vi "PicoScope6000aExampleBlock.vi"() -> ()   [LabVIEW 2016]
uses:
  <vilib>/Waveform/DWDTOps.llb/DWDT Analog to Digital.vi
  PicoScope6000aLib/PicoScope6000aAnalogChannelSettings.ctl
  PicoScope6000aLib/PicoScope6000aDigitalChannelSettings.ctl
panel:
  in  "Digital Channels":T1={"Port 0 Settings "={"Enabled"=FALSE, "Hysteresis"=3, "Threshold Level (Volts)"=[1.0, 1.0, 1.0, 1.0, 1.0, 1.0, 1.0, 1.0]}, "Port 1 Settings"={"Enabled"=FALSE, "Hysteresis"=3, "Threshold Level (Volts)"=[1.0, 1.0, 1.0, 1.0, 1.0, 1.0, 1.0, 1.0]}} {"Port 1 Settings"."Threshold Level (Volts)" format="%#_4p"; "Port 1 Settings"."Hysteresis" items=["PICO_VERY_HIGH_400MV", "PICO_HIGH_200MV", "PICO_NORMAL_100MV", "PICO_LOW_50MV"]; "Port 0 Settings"."Threshold Level (Volts)" format="%#_4p"; "Port 0 Settings"."Hysteresis" items=["PICO_VERY_HIGH_400MV", "PICO_HIGH_200MV", "PICO_NORMAL_100MV", "PICO_LOW_50MV"]}
  in  "Channels":T2={"Channel A Settings "={"Enabled"=TRUE, "Coupling"=1, "Range"=0, "Analogue Offset"=0.0, "BandWidth"=0}, "Channel B Settings "={"Enabled"=FALSE, "Coupling"=1, "Range"=0, "Analogue Offset"=0.0, "BandWidth"=0}, "Channel C Settings "={"Enabled"=FALSE, "Coupling"=1, "Range"=0, "Analogue Offset"=0.0, "BandWidth"=0}, "Channel D Settings "={"Enabled"=FALSE, "Coupling"=1, "Range"=0, "Analogue Offset"=0.0, "BandWidth"=0}, "Channel E Settings "={"Enabled"=FALSE, "Coupling"=1, "Range"=0, "Analogue Offset"=0.0, "BandWidth"=0}, "Channel F Settings "={"Enabled"=FALSE, "Coupling"=1, "Range"=0, "Analogue Offset"=0.0, "BandWidth"=0}, "Channel G Settings "={"Enabled"=FALSE, "Coupling"=1, "Range"=0, "Analogue Offset"=0.0, "BandWidth"=0}, "Channel H Settings "={"Enabled"=FALSE, "Coupling"=1, "Range"=0, "Analogue Offset"=0.0, "BandWidth"=0}} {"Channel H Settings"."BandWidth" items=["Full"=0, "100kHz"=100000, "20kHz"=200000, "1MHz"=1000000, "20MHz"=20000000, "25MHz"=25000000, "50MHz"=50000000, "200MHz"=200000000, "250MHz"=250000000, "500MHz"=500000000]; "Channel H Settings"."Range" items=["10mV"=0, "20mV"=1, "50mV"=2, "100mV"=3, "200mV"=4, "500mV"=5, "1V"=6, "2V"=7, "5V"=8, "10V"=9, "20V"=10, "50V"=11, "100V"=12, "200V"=13, "x10_Probe_100mV"=32, "x10_Probe_200mV"=33, "x10_Probe_500mV"=34, "x10_Probe_1V"=35, "x10_Probe_2V"=36, "x10_Probe_5V"=37, "x10_Probe_10V"=38, "x10_Probe_20V"=39, "x10_Probe_50V"=40, "x10_Probe_100V"=41, "x10_Probe_200V"=42, "x10_Probe_500V"=43, "CURRENT_CLAMP_60A_2A"=10500, "CURRENT_CLAMP_60A_5A"=10501, "CURRENT_CLAMP_60A_10A"=10502, "CURRENT_CLAMP_60A_20A"=10503, "CURRENT_CLAMP_60A_50A"=10504, "CURRENT_CLAMP_60A_60A"=10505, "CURRENT_CLAMP_60A_V2_0_5A"=10600, "CURRENT_CLAMP_60A_V2_1A"=10601, "CURRENT_CLAMP_60A_V2_2A"=10602, "CURRENT_CLAMP_60A_V2_5A"=10603, "CURRENT_CLAMP_60A_V2_10A"=10604, "CURRENT_CLAMP_60A_V2_20A"=10605, "CURRENT_CLAMP_60A_V2_50A"=10606, "CURRENT_CLAMP_60A_V2_60A"=10607, "RESISTANCE_LEAD_NEG5_TO_20OHM"=7000, "RESISTANCE_LEAD_NEG50_TO_200OHM"=7001, "RESISTANCE_LEAD_NEG500_TO_2KOHM"=7002, "RESISTANCE_LEAD_NEG5K_TO_20KOHM"=7003, "RESISTANCE_LEAD_NEG50K_TO_LEAD_200KOHM"=7004, "RESISTANCE_LEAD_NEG500K_TO_LEAD_2MOHM"=7005, "RESISTANCE_LEAD_DIODE_TEST"=7006, "HT_NEG3_TO_5KV"=8950, "HT_NEG3_TO_10KV"=8951, "HT_NEG5_TO_20KV"=8952, "HT_NEG5_TO_50KV"=8953, "HT_NEG5_TO_100KV"=8954, "HT_NEG3_TO_5KV_INVERTED"=8955, "HT_NEG3_TO_10KV_INVERTED"=8956, "HT_NEG5_TO_20KV_INVERTED"=8957, "HT_NEG5_TO_50KV_INVERTED"=8958, "HT_NEG5_TO_100KV_INVERTED"=8959, "TEMPERATURE_NEG50_TO_150DEGC"=9000, "PRESSURE_SENSOR_-100k-150k_PASCALS"=9100, "PRESSURE_SENSOR_-100k_TO_400k_PASCALS"=9101, "PRESSURE_SENSOR_-200k_TO_800k_PASCALS"=9102, "PRESSURE_SENSOR_-400k_TO_1600k_PASCALS"=9103, "PRESSURE_SENSOR_-400k_TO_3400k_PASCALS"=9104, "PRESSURE_SENSOR_-150k_TO_1350k_PASCALS"=9105]; "Channel H Settings"."Coupling" items=["AC"=0, "DC 1M Ohm"=1, "DC 50 Ohm"=50]; "Channel G Settings"."BandWidth" items=["Full"=0, "100kHz"=100000, "20kHz"=200000, "1MHz"=1000000, "20MHz"=20000000, "25MHz"=25000000, "50MHz"=50000000, "200MHz"=200000000, "250MHz"=250000000, "500MHz"=500000000]; "Channel G Settings"."Range" items=["10mV"=0, "20mV"=1, "50mV"=2, "100mV"=3, "200mV"=4, "500mV"=5, "1V"=6, "2V"=7, "5V"=8, "10V"=9, "20V"=10, "50V"=11, "100V"=12, "200V"=13, "x10_Probe_100mV"=32, "x10_Probe_200mV"=33, "x10_Probe_500mV"=34, "x10_Probe_1V"=35, "x10_Probe_2V"=36, "x10_Probe_5V"=37, "x10_Probe_10V"=38, "x10_Probe_20V"=39, "x10_Probe_50V"=40, "x10_Probe_100V"=41, "x10_Probe_200V"=42, "x10_Probe_500V"=43, "CURRENT_CLAMP_60A_2A"=10500, "CURRENT_CLAMP_60A_5A"=10501, "CURRENT_CLAMP_60A_10A"=10502, "CURRENT_CLAMP_60A_20A"=10503, "CURRENT_CLAMP_60A_50A"=10504, "CURRENT_CLAMP_60A_60A"=10505, "CURRENT_CLAMP_60A_V2_0_5A"=10600, "CURRENT_CLAMP_60A_V2_1A"=10601, "CURRENT_CLAMP_60A_V2_2A"=10602, "CURRENT_CLAMP_60A_V2_5A"=10603, "CURRENT_CLAMP_60A_V2_10A"=10604, "CURRENT_CLAMP_60A_V2_20A"=10605, "CURRENT_CLAMP_60A_V2_50A"=10606, "CURRENT_CLAMP_60A_V2_60A"=10607, "RESISTANCE_LEAD_NEG5_TO_20OHM"=7000, "RESISTANCE_LEAD_NEG50_TO_200OHM"=7001, "RESISTANCE_LEAD_NEG500_TO_2KOHM"=7002, "RESISTANCE_LEAD_NEG5K_TO_20KOHM"=7003, "RESISTANCE_LEAD_NEG50K_TO_LEAD_200KOHM"=7004, "RESISTANCE_LEAD_NEG500K_TO_LEAD_2MOHM"=7005, "RESISTANCE_LEAD_DIODE_TEST"=7006, "HT_NEG3_TO_5KV"=8950, "HT_NEG3_TO_10KV"=8951, "HT_NEG5_TO_20KV"=8952, "HT_NEG5_TO_50KV"=8953, "HT_NEG5_TO_100KV"=8954, "HT_NEG3_TO_5KV_INVERTED"=8955, "HT_NEG3_TO_10KV_INVERTED"=8956, "HT_NEG5_TO_20KV_INVERTED"=8957, "HT_NEG5_TO_50KV_INVERTED"=8958, "HT_NEG5_TO_100KV_INVERTED"=8959, "TEMPERATURE_NEG50_TO_150DEGC"=9000, "PRESSURE_SENSOR_-100k-150k_PASCALS"=9100, "PRESSURE_SENSOR_-100k_TO_400k_PASCALS"=9101, "PRESSURE_SENSOR_-200k_TO_800k_PASCALS"=9102, "PRESSURE_SENSOR_-400k_TO_1600k_PASCALS"=9103, "PRESSURE_SENSOR_-400k_TO_3400k_PASCALS"=9104, "PRESSURE_SENSOR_-150k_TO_1350k_PASCALS"=9105]; "Channel G Settings"."Coupling" items=["AC"=0, "DC 1M Ohm"=1, "DC 50 Ohm"=50]; "Channel F Settings"."BandWidth" items=["Full"=0, "100kHz"=100000, "20kHz"=200000, "1MHz"=1000000, "20MHz"=20000000, "25MHz"=25000000, "50MHz"=50000000, "200MHz"=200000000, "250MHz"=250000000, "500MHz"=500000000]; "Channel F Settings"."Range" items=["10mV"=0, "20mV"=1, "50mV"=2, "100mV"=3, "200mV"=4, "500mV"=5, "1V"=6, "2V"=7, "5V"=8, "10V"=9, "20V"=10, "50V"=11, "100V"=12, "200V"=13, "x10_Probe_100mV"=32, "x10_Probe_200mV"=33, "x10_Probe_500mV"=34, "x10_Probe_1V"=35, "x10_Probe_2V"=36, "x10_Probe_5V"=37, "x10_Probe_10V"=38, "x10_Probe_20V"=39, "x10_Probe_50V"=40, "x10_Probe_100V"=41, "x10_Probe_200V"=42, "x10_Probe_500V"=43, "CURRENT_CLAMP_60A_2A"=10500, "CURRENT_CLAMP_60A_5A"=10501, "CURRENT_CLAMP_60A_10A"=10502, "CURRENT_CLAMP_60A_20A"=10503, "CURRENT_CLAMP_60A_50A"=10504, "CURRENT_CLAMP_60A_60A"=10505, "CURRENT_CLAMP_60A_V2_0_5A"=10600, "CURRENT_CLAMP_60A_V2_1A"=10601, "CURRENT_CLAMP_60A_V2_2A"=10602, "CURRENT_CLAMP_60A_V2_5A"=10603, "CURRENT_CLAMP_60A_V2_10A"=10604, "CURRENT_CLAMP_60A_V2_20A"=10605, "CURRENT_CLAMP_60A_V2_50A"=10606, "CURRENT_CLAMP_60A_V2_60A"=10607, "RESISTANCE_LEAD_NEG5_TO_20OHM"=7000, "RESISTANCE_LEAD_NEG50_TO_200OHM"=7001, "RESISTANCE_LEAD_NEG500_TO_2KOHM"=7002, "RESISTANCE_LEAD_NEG5K_TO_20KOHM"=7003, "RESISTANCE_LEAD_NEG50K_TO_LEAD_200KOHM"=7004, "RESISTANCE_LEAD_NEG500K_TO_LEAD_2MOHM"=7005, "RESISTANCE_LEAD_DIODE_TEST"=7006, "HT_NEG3_TO_5KV"=8950, "HT_NEG3_TO_10KV"=8951, "HT_NEG5_TO_20KV"=8952, "HT_NEG5_TO_50KV"=8953, "HT_NEG5_TO_100KV"=8954, "HT_NEG3_TO_5KV_INVERTED"=8955, "HT_NEG3_TO_10KV_INVERTED"=8956, "HT_NEG5_TO_20KV_INVERTED"=8957, "HT_NEG5_TO_50KV_INVERTED"=8958, "HT_NEG5_TO_100KV_INVERTED"=8959, "TEMPERATURE_NEG50_TO_150DEGC"=9000, "PRESSURE_SENSOR_-100k-150k_PASCALS"=9100, "PRESSURE_SENSOR_-100k_TO_400k_PASCALS"=9101, "PRESSURE_SENSOR_-200k_TO_800k_PASCALS"=9102, "PRESSURE_SENSOR_-400k_TO_1600k_PASCALS"=9103, "PRESSURE_SENSOR_-400k_TO_3400k_PASCALS"=9104, "PRESSURE_SENSOR_-150k_TO_1350k_PASCALS"=9105]; "Channel F Settings"."Coupling" items=["AC"=0, "DC 1M Ohm"=1, "DC 50 Ohm"=50]; "Channel E Settings"."BandWidth" items=["Full"=0, "100kHz"=100000, "20kHz"=200000, "1MHz"=1000000, "20MHz"=20000000, "25MHz"=25000000, "50MHz"=50000000, "200MHz"=200000000, "250MHz"=250000000, "500MHz"=500000000]; "Channel E Settings"."Range" items=["10mV"=0, "20mV"=1, "50mV"=2, "100mV"=3, "200mV"=4, "500mV"=5, "1V"=6, "2V"=7, "5V"=8, "10V"=9, "20V"=10, "50V"=11, "100V"=12, "200V"=13, "x10_Probe_100mV"=32, "x10_Probe_200mV"=33, "x10_Probe_500mV"=34, "x10_Probe_1V"=35, "x10_Probe_2V"=36, "x10_Probe_5V"=37, "x10_Probe_10V"=38, "x10_Probe_20V"=39, "x10_Probe_50V"=40, "x10_Probe_100V"=41, "x10_Probe_200V"=42, "x10_Probe_500V"=43, "CURRENT_CLAMP_60A_2A"=10500, "CURRENT_CLAMP_60A_5A"=10501, "CURRENT_CLAMP_60A_10A"=10502, "CURRENT_CLAMP_60A_20A"=10503, "CURRENT_CLAMP_60A_50A"=10504, "CURRENT_CLAMP_60A_60A"=10505, "CURRENT_CLAMP_60A_V2_0_5A"=10600, "CURRENT_CLAMP_60A_V2_1A"=10601, "CURRENT_CLAMP_60A_V2_2A"=10602, "CURRENT_CLAMP_60A_V2_5A"=10603, "CURRENT_CLAMP_60A_V2_10A"=10604, "CURRENT_CLAMP_60A_V2_20A"=10605, "CURRENT_CLAMP_60A_V2_50A"=10606, "CURRENT_CLAMP_60A_V2_60A"=10607, "RESISTANCE_LEAD_NEG5_TO_20OHM"=7000, "RESISTANCE_LEAD_NEG50_TO_200OHM"=7001, "RESISTANCE_LEAD_NEG500_TO_2KOHM"=7002, "RESISTANCE_LEAD_NEG5K_TO_20KOHM"=7003, "RESISTANCE_LEAD_NEG50K_TO_LEAD_200KOHM"=7004, "RESISTANCE_LEAD_NEG500K_TO_LEAD_2MOHM"=7005, "RESISTANCE_LEAD_DIODE_TEST"=7006, "HT_NEG3_TO_5KV"=8950, "HT_NEG3_TO_10KV"=8951, "HT_NEG5_TO_20KV"=8952, "HT_NEG5_TO_50KV"=8953, "HT_NEG5_TO_100KV"=8954, "HT_NEG3_TO_5KV_INVERTED"=8955, "HT_NEG3_TO_10KV_INVERTED"=8956, "HT_NEG5_TO_20KV_INVERTED"=8957, "HT_NEG5_TO_50KV_INVERTED"=8958, "HT_NEG5_TO_100KV_INVERTED"=8959, "TEMPERATURE_NEG50_TO_150DEGC"=9000, "PRESSURE_SENSOR_-100k-150k_PASCALS"=9100, "PRESSURE_SENSOR_-100k_TO_400k_PASCALS"=9101, "PRESSURE_SENSOR_-200k_TO_800k_PASCALS"=9102, "PRESSURE_SENSOR_-400k_TO_1600k_PASCALS"=9103, "PRESSURE_SENSOR_-400k_TO_3400k_PASCALS"=9104, "PRESSURE_SENSOR_-150k_TO_1350k_PASCALS"=9105]; "Channel E Settings"."Coupling" items=["AC"=0, "DC 1M Ohm"=1, "DC 50 Ohm"=50]; "Channel D Settings"."BandWidth" items=["Full"=0, "100kHz"=100000, "20kHz"=200000, "1MHz"=1000000, "20MHz"=20000000, "25MHz"=25000000, "50MHz"=50000000, "200MHz"=200000000, "250MHz"=250000000, "500MHz"=500000000]; "Channel D Settings"."Range" items=["10mV"=0, "20mV"=1, "50mV"=2, "100mV"=3, "200mV"=4, "500mV"=5, "1V"=6, "2V"=7, "5V"=8, "10V"=9, "20V"=10, "50V"=11, "100V"=12, "200V"=13, "x10_Probe_100mV"=32, "x10_Probe_200mV"=33, "x10_Probe_500mV"=34, "x10_Probe_1V"=35, "x10_Probe_2V"=36, "x10_Probe_5V"=37, "x10_Probe_10V"=38, "x10_Probe_20V"=39, "x10_Probe_50V"=40, "x10_Probe_100V"=41, "x10_Probe_200V"=42, "x10_Probe_500V"=43, "CURRENT_CLAMP_60A_2A"=10500, "CURRENT_CLAMP_60A_5A"=10501, "CURRENT_CLAMP_60A_10A"=10502, "CURRENT_CLAMP_60A_20A"=10503, "CURRENT_CLAMP_60A_50A"=10504, "CURRENT_CLAMP_60A_60A"=10505, "CURRENT_CLAMP_60A_V2_0_5A"=10600, "CURRENT_CLAMP_60A_V2_1A"=10601, "CURRENT_CLAMP_60A_V2_2A"=10602, "CURRENT_CLAMP_60A_V2_5A"=10603, "CURRENT_CLAMP_60A_V2_10A"=10604, "CURRENT_CLAMP_60A_V2_20A"=10605, "CURRENT_CLAMP_60A_V2_50A"=10606, "CURRENT_CLAMP_60A_V2_60A"=10607, "RESISTANCE_LEAD_NEG5_TO_20OHM"=7000, "RESISTANCE_LEAD_NEG50_TO_200OHM"=7001, "RESISTANCE_LEAD_NEG500_TO_2KOHM"=7002, "RESISTANCE_LEAD_NEG5K_TO_20KOHM"=7003, "RESISTANCE_LEAD_NEG50K_TO_LEAD_200KOHM"=7004, "RESISTANCE_LEAD_NEG500K_TO_LEAD_2MOHM"=7005, "RESISTANCE_LEAD_DIODE_TEST"=7006, "HT_NEG3_TO_5KV"=8950, "HT_NEG3_TO_10KV"=8951, "HT_NEG5_TO_20KV"=8952, "HT_NEG5_TO_50KV"=8953, "HT_NEG5_TO_100KV"=8954, "HT_NEG3_TO_5KV_INVERTED"=8955, "HT_NEG3_TO_10KV_INVERTED"=8956, "HT_NEG5_TO_20KV_INVERTED"=8957, "HT_NEG5_TO_50KV_INVERTED"=8958, "HT_NEG5_TO_100KV_INVERTED"=8959, "TEMPERATURE_NEG50_TO_150DEGC"=9000, "PRESSURE_SENSOR_-100k-150k_PASCALS"=9100, "PRESSURE_SENSOR_-100k_TO_400k_PASCALS"=9101, "PRESSURE_SENSOR_-200k_TO_800k_PASCALS"=9102, "PRESSURE_SENSOR_-400k_TO_1600k_PASCALS"=9103, "PRESSURE_SENSOR_-400k_TO_3400k_PASCALS"=9104, "PRESSURE_SENSOR_-150k_TO_1350k_PASCALS"=9105]; "Channel D Settings"."Coupling" items=["AC"=0, "DC 1M Ohm"=1, "DC 50 Ohm"=50]; "Channel C Settings"."BandWidth" items=["Full"=0, "100kHz"=100000, "20kHz"=200000, "1MHz"=1000000, "20MHz"=20000000, "25MHz"=25000000, "50MHz"=50000000, "200MHz"=200000000, "250MHz"=250000000, "500MHz"=500000000]; "Channel C Settings"."Range" items=["10mV"=0, "20mV"=1, "50mV"=2, "100mV"=3, "200mV"=4, "500mV"=5, "1V"=6, "2V"=7, "5V"=8, "10V"=9, "20V"=10, "50V"=11, "100V"=12, "200V"=13, "x10_Probe_100mV"=32, "x10_Probe_200mV"=33, "x10_Probe_500mV"=34, "x10_Probe_1V"=35, "x10_Probe_2V"=36, "x10_Probe_5V"=37, "x10_Probe_10V"=38, "x10_Probe_20V"=39, "x10_Probe_50V"=40, "x10_Probe_100V"=41, "x10_Probe_200V"=42, "x10_Probe_500V"=43, "CURRENT_CLAMP_60A_2A"=10500, "CURRENT_CLAMP_60A_5A"=10501, "CURRENT_CLAMP_60A_10A"=10502, "CURRENT_CLAMP_60A_20A"=10503, "CURRENT_CLAMP_60A_50A"=10504, "CURRENT_CLAMP_60A_60A"=10505, "CURRENT_CLAMP_60A_V2_0_5A"=10600, "CURRENT_CLAMP_60A_V2_1A"=10601, "CURRENT_CLAMP_60A_V2_2A"=10602, "CURRENT_CLAMP_60A_V2_5A"=10603, "CURRENT_CLAMP_60A_V2_10A"=10604, "CURRENT_CLAMP_60A_V2_20A"=10605, "CURRENT_CLAMP_60A_V2_50A"=10606, "CURRENT_CLAMP_60A_V2_60A"=10607, "RESISTANCE_LEAD_NEG5_TO_20OHM"=7000, "RESISTANCE_LEAD_NEG50_TO_200OHM"=7001, "RESISTANCE_LEAD_NEG500_TO_2KOHM"=7002, "RESISTANCE_LEAD_NEG5K_TO_20KOHM"=7003, "RESISTANCE_LEAD_NEG50K_TO_LEAD_200KOHM"=7004, "RESISTANCE_LEAD_NEG500K_TO_LEAD_2MOHM"=7005, "RESISTANCE_LEAD_DIODE_TEST"=7006, "HT_NEG3_TO_5KV"=8950, "HT_NEG3_TO_10KV"=8951, "HT_NEG5_TO_20KV"=8952, "HT_NEG5_TO_50KV"=8953, "HT_NEG5_TO_100KV"=8954, "HT_NEG3_TO_5KV_INVERTED"=8955, "HT_NEG3_TO_10KV_INVERTED"=8956, "HT_NEG5_TO_20KV_INVERTED"=8957, "HT_NEG5_TO_50KV_INVERTED"=8958, "HT_NEG5_TO_100KV_INVERTED"=8959, "TEMPERATURE_NEG50_TO_150DEGC"=9000, "PRESSURE_SENSOR_-100k-150k_PASCALS"=9100, "PRESSURE_SENSOR_-100k_TO_400k_PASCALS"=9101, "PRESSURE_SENSOR_-200k_TO_800k_PASCALS"=9102, "PRESSURE_SENSOR_-400k_TO_1600k_PASCALS"=9103, "PRESSURE_SENSOR_-400k_TO_3400k_PASCALS"=9104, "PRESSURE_SENSOR_-150k_TO_1350k_PASCALS"=9105]; "Channel C Settings"."Coupling" items=["AC"=0, "DC 1M Ohm"=1, "DC 50 Ohm"=50]; "Channel B Settings"."BandWidth" items=["Full"=0, "100kHz"=100000, "20kHz"=200000, "1MHz"=1000000, "20MHz"=20000000, "25MHz"=25000000, "50MHz"=50000000, "200MHz"=200000000, "250MHz"=250000000, "500MHz"=500000000]; "Channel B Settings"."Range" items=["10mV"=0, "20mV"=1, "50mV"=2, "100mV"=3, "200mV"=4, "500mV"=5, "1V"=6, "2V"=7, "5V"=8, "10V"=9, "20V"=10, "50V"=11, "100V"=12, "200V"=13, "x10_Probe_100mV"=32, "x10_Probe_200mV"=33, "x10_Probe_500mV"=34, "x10_Probe_1V"=35, "x10_Probe_2V"=36, "x10_Probe_5V"=37, "x10_Probe_10V"=38, "x10_Probe_20V"=39, "x10_Probe_50V"=40, "x10_Probe_100V"=41, "x10_Probe_200V"=42, "x10_Probe_500V"=43, "CURRENT_CLAMP_60A_2A"=10500, "CURRENT_CLAMP_60A_5A"=10501, "CURRENT_CLAMP_60A_10A"=10502, "CURRENT_CLAMP_60A_20A"=10503, "CURRENT_CLAMP_60A_50A"=10504, "CURRENT_CLAMP_60A_60A"=10505, "CURRENT_CLAMP_60A_V2_0_5A"=10600, "CURRENT_CLAMP_60A_V2_1A"=10601, "CURRENT_CLAMP_60A_V2_2A"=10602, "CURRENT_CLAMP_60A_V2_5A"=10603, "CURRENT_CLAMP_60A_V2_10A"=10604, "CURRENT_CLAMP_60A_V2_20A"=10605, "CURRENT_CLAMP_60A_V2_50A"=10606, "CURRENT_CLAMP_60A_V2_60A"=10607, "RESISTANCE_LEAD_NEG5_TO_20OHM"=7000, "RESISTANCE_LEAD_NEG50_TO_200OHM"=7001, "RESISTANCE_LEAD_NEG500_TO_2KOHM"=7002, "RESISTANCE_LEAD_NEG5K_TO_20KOHM"=7003, "RESISTANCE_LEAD_NEG50K_TO_LEAD_200KOHM"=7004, "RESISTANCE_LEAD_NEG500K_TO_LEAD_2MOHM"=7005, "RESISTANCE_LEAD_DIODE_TEST"=7006, "HT_NEG3_TO_5KV"=8950, "HT_NEG3_TO_10KV"=8951, "HT_NEG5_TO_20KV"=8952, "HT_NEG5_TO_50KV"=8953, "HT_NEG5_TO_100KV"=8954, "HT_NEG3_TO_5KV_INVERTED"=8955, "HT_NEG3_TO_10KV_INVERTED"=8956, "HT_NEG5_TO_20KV_INVERTED"=8957, "HT_NEG5_TO_50KV_INVERTED"=8958, "HT_NEG5_TO_100KV_INVERTED"=8959, "TEMPERATURE_NEG50_TO_150DEGC"=9000, "PRESSURE_SENSOR_-100k-150k_PASCALS"=9100, "PRESSURE_SENSOR_-100k_TO_400k_PASCALS"=9101, "PRESSURE_SENSOR_-200k_TO_800k_PASCALS"=9102, "PRESSURE_SENSOR_-400k_TO_1600k_PASCALS"=9103, "PRESSURE_SENSOR_-400k_TO_3400k_PASCALS"=9104, "PRESSURE_SENSOR_-150k_TO_1350k_PASCALS"=9105]; "Channel B Settings"."Coupling" items=["AC"=0, "DC 1M Ohm"=1, "DC 50 Ohm"=50]; "Channel A Settings"."Range" items=["10mV"=0, "20mV"=1, "50mV"=2, "100mV"=3, "200mV"=4, "500mV"=5, "1V"=6, "2V"=7, "5V"=8, "10V"=9, "20V"=10, "50V"=11, "100V"=12, "200V"=13, "x10_Probe_100mV"=32, "x10_Probe_200mV"=33, "x10_Probe_500mV"=34, "x10_Probe_1V"=35, "x10_Probe_2V"=36, "x10_Probe_5V"=37, "x10_Probe_10V"=38, "x10_Probe_20V"=39, "x10_Probe_50V"=40, "x10_Probe_100V"=41, "x10_Probe_200V"=42, "x10_Probe_500V"=43, "CURRENT_CLAMP_60A_2A"=10500, "CURRENT_CLAMP_60A_5A"=10501, "CURRENT_CLAMP_60A_10A"=10502, "CURRENT_CLAMP_60A_20A"=10503, "CURRENT_CLAMP_60A_50A"=10504, "CURRENT_CLAMP_60A_60A"=10505, "CURRENT_CLAMP_60A_V2_0_5A"=10600, "CURRENT_CLAMP_60A_V2_1A"=10601, "CURRENT_CLAMP_60A_V2_2A"=10602, "CURRENT_CLAMP_60A_V2_5A"=10603, "CURRENT_CLAMP_60A_V2_10A"=10604, "CURRENT_CLAMP_60A_V2_20A"=10605, "CURRENT_CLAMP_60A_V2_50A"=10606, "CURRENT_CLAMP_60A_V2_60A"=10607, "RESISTANCE_LEAD_NEG5_TO_20OHM"=7000, "RESISTANCE_LEAD_NEG50_TO_200OHM"=7001, "RESISTANCE_LEAD_NEG500_TO_2KOHM"=7002, "RESISTANCE_LEAD_NEG5K_TO_20KOHM"=7003, "RESISTANCE_LEAD_NEG50K_TO_LEAD_200KOHM"=7004, "RESISTANCE_LEAD_NEG500K_TO_LEAD_2MOHM"=7005, "RESISTANCE_LEAD_DIODE_TEST"=7006, "HT_NEG3_TO_5KV"=8950, "HT_NEG3_TO_10KV"=8951, "HT_NEG5_TO_20KV"=8952, "HT_NEG5_TO_50KV"=8953, "HT_NEG5_TO_100KV"=8954, "HT_NEG3_TO_5KV_INVERTED"=8955, "HT_NEG3_TO_10KV_INVERTED"=8956, "HT_NEG5_TO_20KV_INVERTED"=8957, "HT_NEG5_TO_50KV_INVERTED"=8958, "HT_NEG5_TO_100KV_INVERTED"=8959, "TEMPERATURE_NEG50_TO_150DEGC"=9000, "PRESSURE_SENSOR_-100k-150k_PASCALS"=9100, "PRESSURE_SENSOR_-100k_TO_400k_PASCALS"=9101, "PRESSURE_SENSOR_-200k_TO_800k_PASCALS"=9102, "PRESSURE_SENSOR_-400k_TO_1600k_PASCALS"=9103, "PRESSURE_SENSOR_-400k_TO_3400k_PASCALS"=9104, "PRESSURE_SENSOR_-150k_TO_1350k_PASCALS"=9105]; "Channel A Settings"."BandWidth" items=["Full"=0, "100kHz"=100000, "20kHz"=200000, "1MHz"=1000000, "20MHz"=20000000, "25MHz"=25000000, "50MHz"=50000000, "200MHz"=200000000, "250MHz"=250000000, "500MHz"=500000000]; "Channel A Settings"."Coupling" items=["AC"=0, "DC 1M Ohm"=1, "DC 50 Ohm"=50]}
  in  "Trigger Settings":T3={"Trigger Enabled"=FALSE, "Trigger Threshold (Volts)"=0.0, "Trigger Direction"=2, "Trigger Delay (samples)"=0, "Auto Trigger Time (us)"=1000, "Trigger Source"=0} {"Trigger Source" items=["Channel A"=0, "Channel B"=1, "Channel C"=2, "Channel D"=3, "Channel E"=4, "Channel F"=5, "Channel G"=6, "Channel H"=7, "Port 0"=128, "Port 1"=129, "Trigger AUX"=1001]; "Trigger Direction" items=["Above", "Below", "Rising", "Falling", "Rising or Falling"]; "Trigger Threshold (Volts)" format="%#_6p"}
  in  "Buffer and Transfer Settings":T4={"startIndex"=0, "Samples"=100000000, "Down Sample Ratio"=10, "Down-Sample Mode"=2} {"Down-Sample Mode" items=["None"=2147483648, "Aggregate"=1, "Decimate"=2, "Average"=4]; "Down Sample Ratio" step=1; "Samples" format="%_6p"}
  in  "Acquisition Settings":T5={"preTriggerSamples"=0, "postTriggerSamples"=1000000000, "timebase"=2} {"postTriggerSamples" format="%_6p"; "preTriggerSamples" format="%_6p"}
  out "Properties Panel":T6={"Sample Frequency"=1250000000.0, "Sample Rate"=8e-10, "Max Samples Available"=4294966784, "Number of Samples"=10000000, "Total Capture Time (sec) "=0.008, "Max Total Capture Time Available (sec)"=3.4359734272} {"Max Total Capture Time Available (sec)" format="%.3p"; "Sample Frequency" format="%.6p"; "Sample Rate" format="%.3p"; "Max Samples Available" format="%_6p"; "Total Capture Time (sec)" format="%.3p"}
  out "Port 0":digitalwaveform(graph)={"t0"=timestamp(0 s since 1904-01-01), "dt"=8e-09, "Y"={"transitions"=[], "data"=[]}}
  in  "stop":bool
  out "Analog Channels":cluster{i32, dbl, "Data (Volts)":dbl[]}[](graph)=[{0, 8e-09, "Data (Volts)"=[]}, {0, 8e-09, "Data (Volts)"=[]}, {0, 8e-09, "Data (Volts)"=[]}, {0, 8e-09, "Data (Volts)"=[]}, {0, 8e-09, "Data (Volts)"=[]}, {0, 8e-09, "Data (Volts)"=[]}, {0, 8e-09, "Data (Volts)"=[]}, {0, 8e-09, "Data (Volts)"=[]}]
  out "overflow":i16 format="%08b"
  out "Device Info":T7={"PICO_DRIVER_VERSION"="", "PICO_USB_VERSION"="", "PICO_HARDWARE_VERSION"="", "PICO_VARIANT_INFO"="", "PICO_BATCH_AND_SERIAL"="", "PICO_CAL_DATE"="", "PICO_KERNEL_VERSION"="", "PICO_DIGITAL_HARDWARE_VERSION"="", "PICO_ANALOGUE_HARDWARE_VERSION"="", "PICO_FIRMWARE_VERSION_1"="", "PICO_FIRMWARE_VERSION_2"="", "PICO_IPP_VERSION"="", "PICO_DRIVER_PATH"="", "PICO_FIRMWARE_VERSION_3"="", "PICO_FRONT_PANEL_FIRMWARE_VERSION"="", "Number of Channels"=0, "MSO"=TRUE}
  out "Pico 6000a Units":string
  in  "Resolution":u32(ring) items=["8-bit"=0, "12-bit"=1, "14-bit"=2, "15-bit"=3, "16-bit"=4, "10-bit"=10]
  in  "Serial Number":string
  in  "Use Serial Number":bool
  in  "error in (no error)":errorcluster
  # "Please Ensure you set the \"Range\"(Probe type) before running the VI"
  # "D8-D15"
  # "DO-D7"
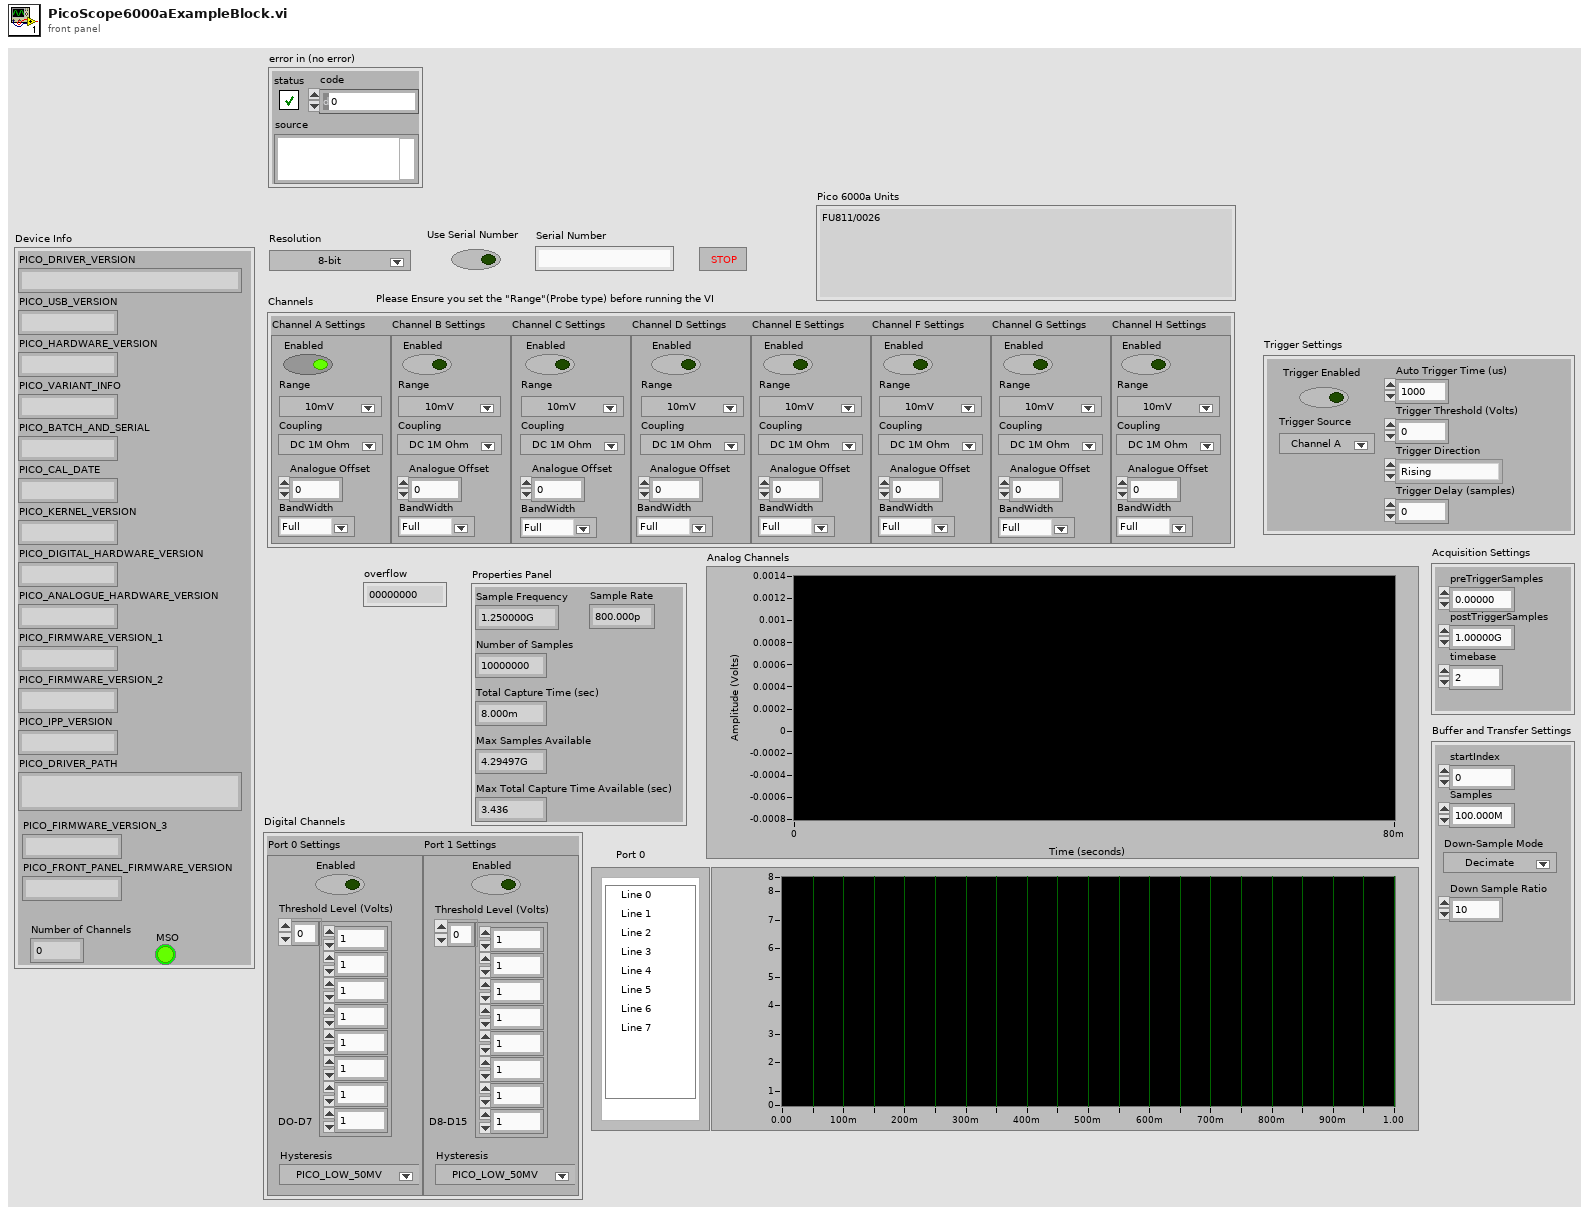
[diagram p1: front panel]
types:
  T1 = typedef "PicoScope6000aDigitalChannelSettings.ctl" = cluster{"Port 0 Settings ":cluster{"Enabled":bool, "Hysteresis":u32, "Threshold Level (Volts)":dbl[]}, "Port 1 Settings":cluster{"Enabled":bool, "Hysteresis":u32, "Threshold Level (Volts)":dbl[]}}
  T2 = typedef "PicoScope6000aAnalogChannelSettings.ctl" = cluster{"Channel A Settings ":cluster{"Enabled":bool, "Coupling":i16, "Range":u16, "Analogue Offset":dbl, "BandWidth":u32}, "Channel B Settings ":cluster{"Enabled":bool, "Coupling":i16, "Range":u16, "Analogue Offset":dbl, "BandWidth":u32}, "Channel C Settings ":cluster{"Enabled":bool, "Coupling":i16, "Range":u16, "Analogue Offset":dbl, "BandWidth":u32}, "Channel D Settings ":cluster{"Enabled":bool, "Coupling":i16, "Range":u16, "Analogue Offset":dbl, "BandWidth":u32}, "Channel E Settings ":cluster{"Enabled":bool, "Coupling":i16, "Range":u16, "Analogue Offset":dbl, "BandWidth":u32}, "Channel F Settings ":cluster{"Enabled":bool, "Coupling":i16, "Range":u16, "Analogue Offset":dbl, "BandWidth":u32}, "Channel G Settings ":cluster{"Enabled":bool, "Coupling":i16, "Range":u16, "Analogue Offset":dbl, "BandWidth":u32}, "Channel H Settings ":cluster{"Enabled":bool, "Coupling":i16, "Range":u16, "Analogue Offset":dbl, "BandWidth":u32}}
  T3 = cluster{"Trigger Enabled":bool, "Trigger Threshold (Volts)":dbl, "Trigger Direction":u16, "Trigger Delay (samples)":u64, "Auto Trigger Time (us)":u32, "Trigger Source":u32}
  T4 = cluster{"startIndex":u64, "Samples":u64, "Down Sample Ratio":u64, "Down-Sample Mode":u32}
  T5 = cluster{"preTriggerSamples":u64, "postTriggerSamples":u64, "timebase":u32}
  T6 = cluster{"Sample Frequency":dbl, "Sample Rate":dbl, "Max Samples Available":u64, "Number of Samples":u64, "Total Capture Time (sec) ":dbl, "Max Total Capture Time Available (sec)":dbl}
  T7 = cluster{"PICO_DRIVER_VERSION":string, "PICO_USB_VERSION":string, "PICO_HARDWARE_VERSION":string, "PICO_VARIANT_INFO":string, "PICO_BATCH_AND_SERIAL":string, "PICO_CAL_DATE":string, "PICO_KERNEL_VERSION":string, "PICO_DIGITAL_HARDWARE_VERSION":string, "PICO_ANALOGUE_HARDWARE_VERSION":string, "PICO_FIRMWARE_VERSION_1":string, "PICO_FIRMWARE_VERSION_2":string, "PICO_IPP_VERSION":string, "PICO_DRIVER_PATH":string, "PICO_FIRMWARE_VERSION_3":string, "PICO_FRONT_PANEL_FIRMWARE_VERSION":string, "Number of Channels":i16, "MSO":bool}
  T8 = cluster{"Channel A Buffer":i16[], "Channel B Buffer":i16[], "Channel C Buffer":i16[], "Channel D Buffer":i16[], "Channel E Buffer":i16[], "Channel F Buffer":i16[], "Channel G Buffer":i16[], "Channel H Buffer":i16[], "Port 0 Buffer":i16[], "Port 1 Buffer":i16[]}
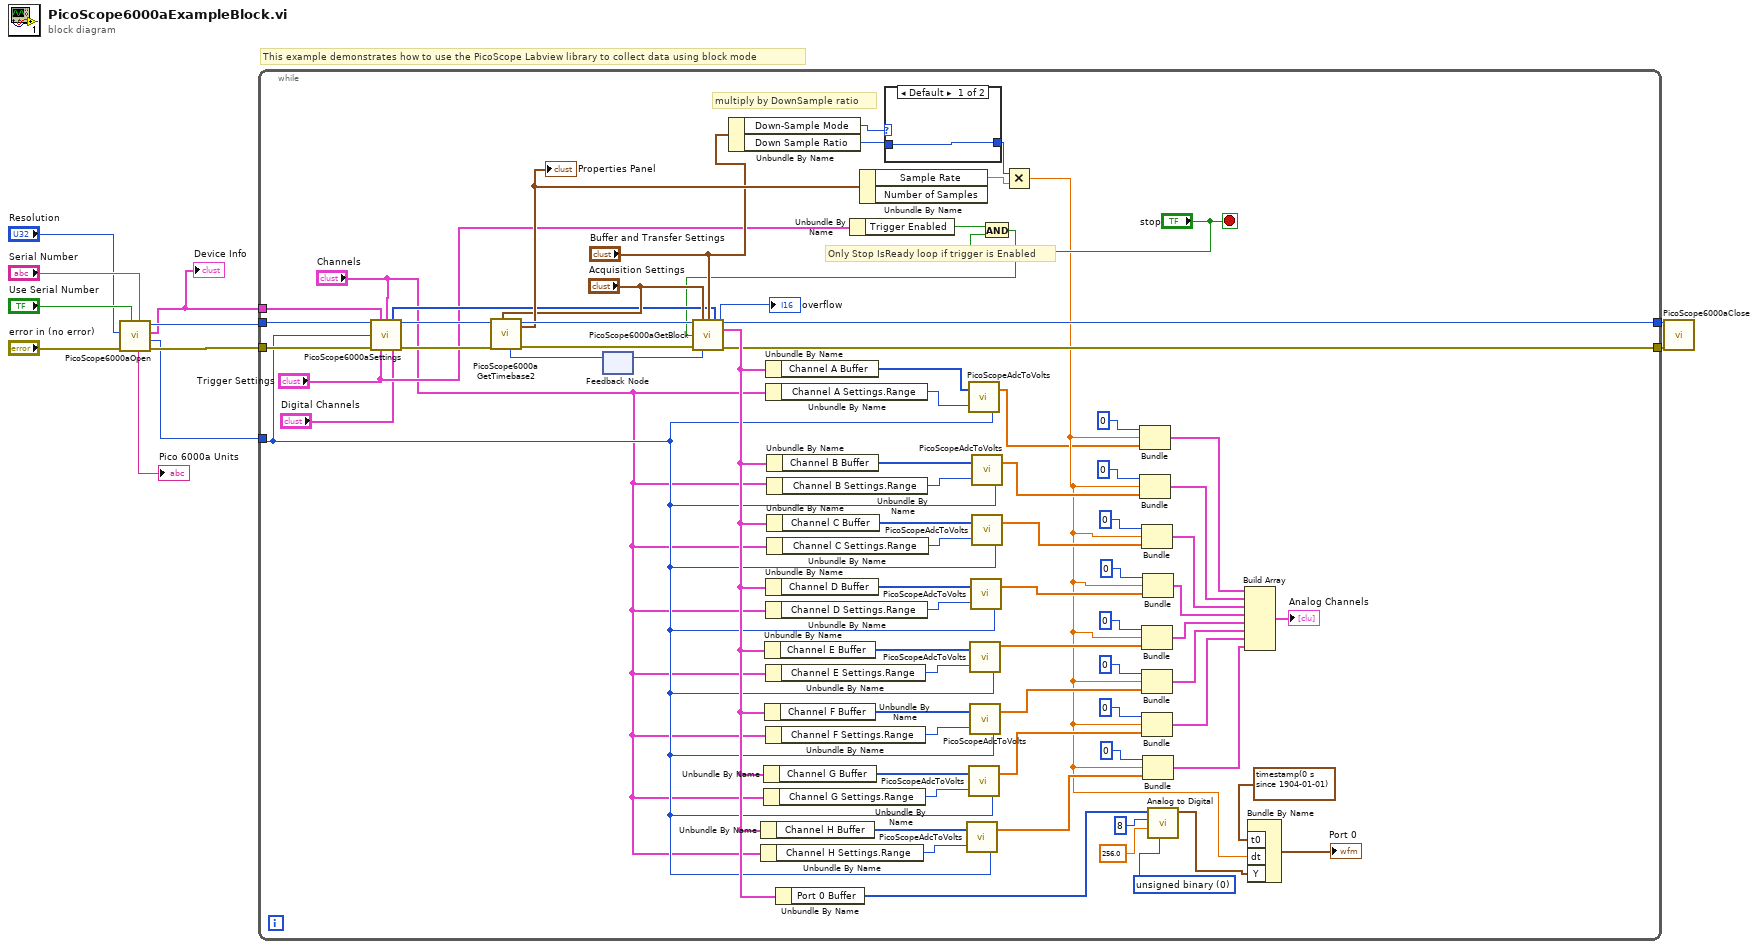
[diagram p0: block diagram]
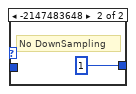
[diagram p2: hidden frame]
diagram:
  # "This example demonstrates how to use the PicoScope Labview library to collect data using block mode"
  n1 = call "PicoScope6000aOpen.vi"("Serial Number"="Serial Number", "Use Serial Number"="Use Serial Number", "error in (no error)"="error in (no error)", "Resolution"="Resolution") -> ("error out"=w7:errorcluster, "Max ADC value"=w2:i16, "Device Info"=w1:T7, "handle out"=w8:i16, "Pico 6000a Units"=→"Pico 6000a Units":string)  [unwired: 2 in, 1 out]
  "Device Info" <- w1
  n2 = while {
    tunnel: w1 -> [w85]
    tunnel: w2 -> [w26]
    tunnel: w8 -> [w88]
    tunnel: [w86] -> w6
    tunnel: w7 -> [w87]
    tunnel: [w38] -> w5
    stop <- "stop" stop-if-true
    w43 = u16 0 items=["unsigned binary", "offset binary", "2's complement"] ("data format (offset binary)")
    # "multiply by DownSample ratio"
    # "Only Stop IsReady loop if trigger is Enabled"
    n3 = call "PicoScope6000aSettings.vi"("handle in"=w88, "Device Info"=w85, "Channels"="Channels", "Max ADC value"=w26, "error in (no error)"=w87, "Trigger Settings"="Trigger Settings", "Digital Channels"="Digital Channels") -> ("Enabled array"=w17:i16[], "handle out"=w34:i16, "error out"=w37:errorcluster)  [unwired: 6 in]
    n4 = feedback #1() -> (w32:u64)  [unwired: 1 in]
    n5 = call "PicoScope6000aGetTimebase2.vi"("Number of Samples"=w32, "Acquisition Settings"="Acquisition Settings", "error in (no error)"=w37, "handle in"=w34) -> ("error out"=w36:errorcluster, "handle out"=w35:i16, "Properties Panel"=w25:T6)  [unwired: 5 in]
    "Properties Panel" <- w25
    n6 = Unbundle By Name("Buffer and Transfer Settings") -> ("Down-Sample Mode"=w24:u32, "Down Sample Ratio"=w23:u64)
    n7 = Unbundle By Name("Channels") -> ("Channel H Settings.Range"=w63:u16)
    n8 = Unbundle By Name("Channels") -> ("Channel G Settings.Range"=w64:u16)
    n9 = Unbundle By Name("Channels") -> ("Channel A Settings.Range"=w82:u16)
    n10 = Unbundle By Name("Channels") -> ("Channel D Settings.Range"=w70:u16)
    n11 = Unbundle By Name("Channels") -> ("Channel E Settings.Range"=w68:u16)
    n12 = Unbundle By Name("Channels") -> ("Channel F Settings.Range"=w66:u16)
    n13 = Unbundle By Name("Channels") -> ("Channel B Settings.Range"=w78:u16)
    n14 = Unbundle By Name("Channels") -> ("Channel C Settings.Range"=w72:u16)
    n15 = Unbundle By Name("Trigger Settings") -> ("Trigger Enabled"=w28:bool)
    n16 = Unbundle By Name(w25) -> ("Sample Rate"=w21:dbl)  [unwired: 1 out]
    n17 = case shown="Default" w24 {
      tunnel: [w89 u64 1 ("Down Sample Ratio")] -> w20
      tunnel: w23 -> [w89 _]
      frame Default {
      }
      frame -2147483648 {
        # "No DownSampling"
      }
    }
    n18 = And(x=w28, y="stop") -> (x .and. y?=w16:bool)
    n19 = call "PicoScope6000aGetBlock.vi"("handle in"=w35, "Acquisition Settings"="Acquisition Settings", "Buffer and Transfer Settings"="Buffer and Transfer Settings", "enabled array"=w17, "stop IsReady"=w16, "error in (no error)"=w36) -> ("handle out"=w86:i16, "Buffers (Max or non-aggregated)"=w39:T8, "noOfSamples"=w33:u64, "overflow"=→"overflow":i16, "error out"=w38:errorcluster)  [unwired: 4 in, 1 out]
    n20 = feedback-in #1(w33) -> ()
    n21 = Unbundle By Name(w39) -> ("Channel H Buffer"=w41:i16[])
    n22 = Unbundle By Name(w39) -> ("Channel G Buffer"=w65:i16[])
    n23 = Unbundle By Name(w39) -> ("Channel E Buffer"=w69:i16[])
    n24 = Unbundle By Name(w39) -> ("Channel F Buffer"=w67:i16[])
    n25 = Unbundle By Name(w39) -> ("Channel A Buffer"=w83:i16[])
    n26 = Unbundle By Name(w39) -> ("Channel D Buffer"=w71:i16[])
    n27 = Unbundle By Name(w39) -> ("Channel B Buffer"=w79:i16[])
    n28 = Unbundle By Name(w39) -> ("Channel C Buffer"=w73:i16[])
    n29 = Unbundle By Name(w39) -> ("Port 0 Buffer"=w40:i16[])
    n30 = call "PicoScopeAdcToVolts.vi"("Max_adc"=w26, "Range Index"=w63, "Data"=w41) -> ("Data"=w58:dbl[])
    n31 = call "PicoScopeAdcToVolts.vi"("Max_adc"=w26, "Range Index"=w82, "Data"=w83) -> ("Data"=w14:dbl[])
    n32 = call "PicoScopeAdcToVolts.vi"("Max_adc"=w26, "Range Index"=w64, "Data"=w65) -> ("Data"=w52:dbl[])
    n33 = call "PicoScopeAdcToVolts.vi"("Max_adc"=w26, "Range Index"=w68, "Data"=w69) -> ("Data"=w55:dbl[])
    n34 = call "PicoScopeAdcToVolts.vi"("Max_adc"=w26, "Range Index"=w66, "Data"=w67) -> ("Data"=w51:dbl[])
    n35 = call "PicoScopeAdcToVolts.vi"("Max_adc"=w26, "Range Index"=w70, "Data"=w71) -> ("Data"=w56:dbl[])
    n36 = call "PicoScopeAdcToVolts.vi"("Max_adc"=w26, "Range Index"=w78, "Data"=w79) -> ("Data"=w77:dbl[])
    n37 = call "PicoScopeAdcToVolts.vi"("Max_adc"=w26, "Range Index"=w72, "Data"=w73) -> ("Data"=w57:dbl[])
    n38 = Multiply(x=w20, y=w21) -> (x*y=w22:dbl)
    n39 = Bundle(0, w22, "Data"=w14) -> (w76:cluster{i32, dbl, "Data":dbl[]})  [unwired: 1 in]
    n40 = Bundle(0, w22, "Data"=w77) -> (w75:cluster{i32, dbl, "Data":dbl[]})  [unwired: 1 in]
    n41 = Bundle(0, w22, "Data"=w57) -> (w50:cluster{i32, dbl, "Data":dbl[]})  [unwired: 1 in]
    n42 = Bundle(0, w22, "Data"=w55) -> (w48:cluster{i32, dbl, "Data":dbl[]})  [unwired: 1 in]
    n43 = Bundle(0, w22, "Data"=w51) -> (w47:cluster{i32, dbl, "Data":dbl[]})  [unwired: 1 in]
    n44 = Bundle(0, w22, "Data"=w52) -> (w46:cluster{i32, dbl, "Data":dbl[]})  [unwired: 1 in]
    n45 = Bundle(0, w22, "Data"=w56) -> (w49:cluster{i32, dbl, "Data":dbl[]})  [unwired: 1 in]
    n46 = Bundle(0, w22, "Data"=w58) -> (w45:cluster{i32, dbl, "Data":dbl[]})  [unwired: 1 in]
    n47 = call-poly <vilib>:"Analog to Digital.vi"("data format (offset binary)"=w43, "full-scale range (pk-pk)"=256.0, "resolution (16 bit)"=8, "analog waveform"=w40) -> ("digital waveform"=w29:digitalwaveform)  [unwired: 4 in, 3 out]
    n48 = Build Array(w76, w75, w50, w49, w48, w47, w46, w45) -> (→"Analog Channels":cluster{i32, dbl, "Data":dbl[]}[])
    n49 = Bundle By Name("t0"=timestamp(0 s since 1904-01-01), "dt"=w22, "Y"=w29) -> (→"Port 0":digitalwaveform)  [unwired: 1 in]
  }
  n50 = call "PicoScope6000aClose.vi"("error in (no error)"=w5, "handle in"=w6) -> ()  [unwired: 8 in, 2 out]
